vi "TLMB_Snapshot_Status.vi"(0 "GEA2 Reference In":refnum<k24>, 5 "Stand Alone?":bool, 11 "Error In":errorcluster) -> (4 "GEA2 Reference Out":refnum<k24>, 6 "Current Index":u16, 8 "Count":u16, 10 "Overwrite Count":u16, 15 "Error Out":errorcluster)   [LabVIEW 2021, in "TLMB.lvlib"]
uses:
  Projects/TLMB.lvlib
  D:/Common/LabVIEW GEA2 Toolkit/source/GEA3 DLL Source/GeaCommunication.dll
  Common/LabVIEW GEA2 Toolkit/source/GEA3 DLL Source/GeaCommunication.dll
  Common/LabVIEW GEA2 Toolkit/GEA3/type defs/Source_Destination.ctl
  Common/LabVIEW GEA2 Toolkit/GEA3/type defs/ERD Read Data In.ctl
  Common/LabVIEW GEA2 Toolkit/GEA3/library/GEA2_Toolkit.lvlib
panel:
  out "Reserved":u16
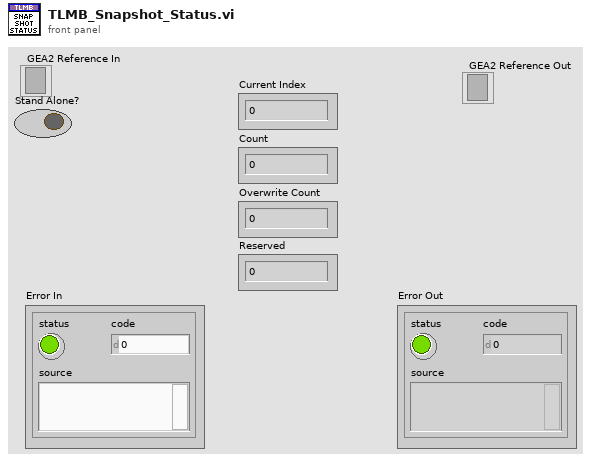
[diagram p1: front panel]
types:
  T1 = typedef "ERD Read Data In.ctl" = cluster{"ERD Number":u16, "Data Type":enum16{"string", "boolean", "uint8_t", "uint16_t", "uint32_t", "uint64_t", "int8_t", "int16_t", "int32_t", "int64_t"}}
  T2 = typedef "Source_Destination.ctl" = cluster{"Source":u8, "Destination":u8}
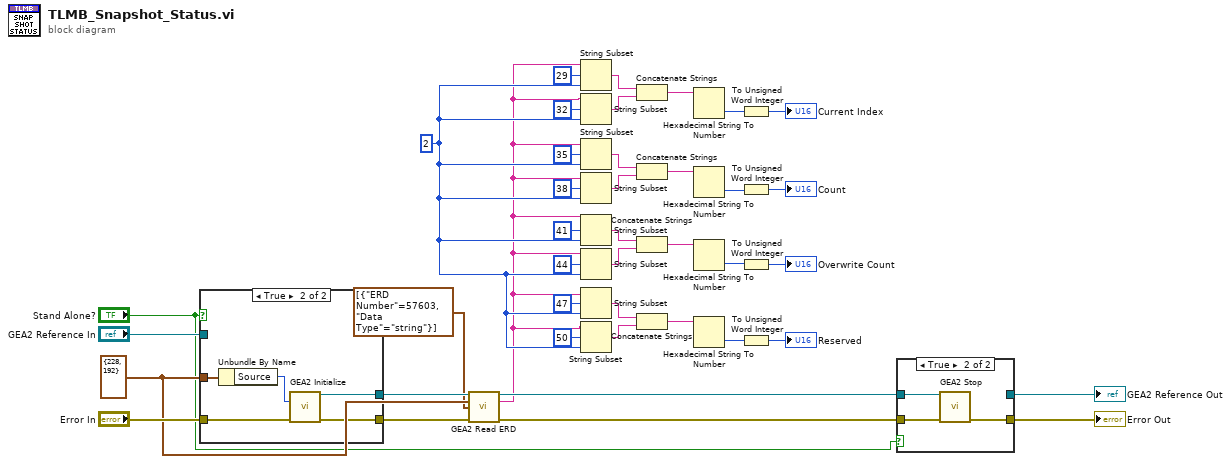
[diagram p0: block diagram]
diagram:
  w30 = 2 ("length (rest)")
  w37 = T2 {"Source"=228, "Destination"=192} ("GEA Inputs")
  n1 = case shown="True" "Stand Alone?" {
    tunnel: "Error In" -> [w42 w48]
    tunnel: [w42 w47] -> w38
    tunnel: "GEA2 Reference In" -> [w43 _]
    tunnel: [w43 w46] -> w40
    tunnel: w37 -> [_ w44]
    frame False {
    }
    frame True {
      n2 = Unbundle By Name(w44) -> ("Source"=w45:u8)
      n3 = call "GEA2 Initialize.vi"("Source Address"=w45, "error in"=w48) -> ("GEA2 Reference Out"=w46:refnum<k24>, "error out"=w47:errorcluster)  [unwired: 11 in, 1 out]
    }
  }
  n4 = call "GEA2 Read ERD.vi"("GEA2 Reference In"=w40, "GEA Inputs"=w37, "Read ERD List"=T1[] [{"ERD Number"=57603, "Data Type"=enum."string"}], "Error In"=w38) -> ("GEA2 Reference Out"=w33:refnum<k24>, "Raw Data Out"=w29:string, "Error Out"=w32:errorcluster)  [unwired: 8 in, 1 out]
  n5 = String Subset(string=w29, offset (0)=29, length (rest)=w30) -> (substring=w20:string)
  n6 = String Subset(string=w29, offset (0)=32, length (rest)=w30) -> (substring=w19:string)
  n7 = String Subset(string=w29, offset (0)=35, length (rest)=w30) -> (substring=w18:string)
  n8 = String Subset(string=w29, offset (0)=38, length (rest)=w30) -> (substring=w17:string)
  n9 = String Subset(string=w29, offset (0)=41, length (rest)=w30) -> (substring=w16:string)
  n10 = String Subset(string=w29, offset (0)=44, length (rest)=w30) -> (substring=w15:string)
  n11 = String Subset(string=w29, offset (0)=47, length (rest)=w30) -> (substring=w14:string)
  n12 = String Subset(string=w29, offset (0)=50, length (rest)=w30) -> (substring=w13:string)
  n13 = Concatenate Strings(w20, w19) -> (w12:string)
  n14 = Concatenate Strings(w18, w17) -> (w11:string)
  n15 = Concatenate Strings(w16, w15) -> (w10:string)
  n16 = Concatenate Strings(w14, w13) -> (w9:string)
  n17 = Hexadecimal String To Number(string=w12) -> (number=w8:u32)  [unwired: 2 in, 1 out]
  n18 = Hexadecimal String To Number(string=w11) -> (number=w7:u32)  [unwired: 2 in, 1 out]
  n19 = Hexadecimal String To Number(string=w10) -> (number=w6:u32)  [unwired: 2 in, 1 out]
  n20 = Hexadecimal String To Number(string=w9) -> (number=w5:u32)  [unwired: 2 in, 1 out]
  n21 = To Unsigned Word Integer(number=w8) -> (unsigned 16bit integer=→"Current Index":u16)
  n22 = To Unsigned Word Integer(number=w7) -> (unsigned 16bit integer=→"Count":u16)
  n23 = To Unsigned Word Integer(number=w6) -> (unsigned 16bit integer=→"Overwrite Count":u16)
  n24 = To Unsigned Word Integer(number=w5) -> (unsigned 16bit integer=→"Reserved":u16)
  n25 = case shown="True" "Stand Alone?" {
    tunnel: [w49 w53] -> w34
    tunnel: w33 -> [w50 w52]
    tunnel: [w50 _] -> w35
    tunnel: w32 -> [w49 w51]
    frame False {
    }
    frame True {
      n26 = call "GEA2 Stop.vi"("GEA2 Reference In"=w52, "Error In"=w51) -> ("Error Out"=w53:errorcluster)  [unwired: 13 in]
    }
  }
  "Error Out" <- w34
  "GEA2 Reference Out" <- w35
